vi "Begin.vi"(11 "Image Size":T6=enum."160x120") -> (0 "error out":errorcluster)   [LabVIEW 2011]
doc: "Called before other user functions, this VI is expected to open initial I/O refnums, load in file data, and do all program initialization. Notice that the <B>error out</B> terminal is simply used for data flow. Wiring it to other structures or subVIs ensures that this VI runs first."
uses:
  <vilib>/Rock Robotics/WPI/Camera/WPI_CameraImageSize.ctl
  <vilib>/Rock Robotics/SystemInterfaces/Typedef/FPGA_TypedefDigitalModule.ctl
  <vilib>/Rock Robotics/SystemInterfaces/CounterEncoderSourceConvertion/FPGA_CounterEncoderSourceConvertionLVSourceType.ctl
  <vilib>/Rock Robotics/SystemInterfaces/DIO/FPGA_DIODigitalSourceChannel.ctl
  <vilib>/Rock Robotics/SystemInterfaces/AnalogTrigger/FPGA_AnalogTriggerIndex.ctl
  <vilib>/Rock Robotics/SystemInterfaces/AnalogTrigger/FPGA_AnalogTriggerOutType.ctl
  <vilib>/Rock Robotics/WPI/Joystick/WPI_JoystickDeviceEnum.ctl
  <vilib>/Rock Robotics/WPI/Camera/WPI_CameraWhite Balance Values.ctl
  <vilib>/Rock Robotics/WPI/Camera/WPI_CameraExposure Values.ctl
  <vilib>/Rock Robotics/WPI/Camera/WPI_CameraFrameRate.ctl
  <vilib>/Rock Robotics/SystemInterfaces/DIO/FPGA_DIOPWMChannel.ctl
  <vilib>/Rock Robotics/WPI/Solenoid/WPI_SolenoidChannel.ctl
  <vilib>/Rock Robotics/SystemInterfaces/DIO/FPGA_DIORelayChannel.ctl
  <vilib>/Rock Robotics/SystemInterfaces/DIO/FPGA_DIOChannel.ctl
  <vilib>/Rock Robotics/SystemInterfaces/AI/FPGA_AIChannel.ctl
  <vilib>/Rock Robotics/WPI/Encoder/WPI_EncoderType.ctl
  <vilib>/Rock Robotics/WPI/RobotDrive/WPI_RobotDriveOpen2MotorWithVictor.vi
  <vilib>/Rock Robotics/WPI/Solenoid/WPI_SolenoidOpenSingle.vi
  <vilib>/Rock Robotics/WPI/Compressor/WPI_CompressorGetSetRefNum.vi
panel:
  in  "BSource 2":T1={"DevStatus"={"status"=FALSE, "code"=0, "source"=""}, "AnalogTriggerMode?"=FALSE, "DigitalMode"={"Digital Module"=enum."Digital Module 1", "DIO Channel"=enum."Disabled"}, "AnalogTriggerMode"={"AnalogTriggerIndex"=enum."Trig 0", "OutputType"=enum."InWindow"}}
  in  "ASource 2":T1={"DevStatus"={"status"=FALSE, "code"=0, "source"=""}, "AnalogTriggerMode?"=FALSE, "DigitalMode"={"Digital Module"=enum."Digital Module 1", "DIO Channel"=enum."Disabled"}, "AnalogTriggerMode"={"AnalogTriggerIndex"=enum."Trig 0", "OutputType"=enum."InWindow"}}
  in  "BSource":T1={"DevStatus"={"status"=FALSE, "code"=0, "source"=""}, "AnalogTriggerMode?"=FALSE, "DigitalMode"={"Digital Module"=enum."Digital Module 1", "DIO Channel"=enum."Disabled"}, "AnalogTriggerMode"={"AnalogTriggerIndex"=enum."Trig 0", "OutputType"=enum."InWindow"}}
  in  "ASource":T1={"DevStatus"={"status"=FALSE, "code"=0, "source"=""}, "AnalogTriggerMode?"=FALSE, "DigitalMode"={"Digital Module"=enum."Digital Module 1", "DIO Channel"=enum."Disabled"}, "AnalogTriggerMode"={"AnalogTriggerIndex"=enum."Trig 0", "OutputType"=enum."InWindow"}}
  in  "Pressure Switch Digital Module (Module 1)":T2
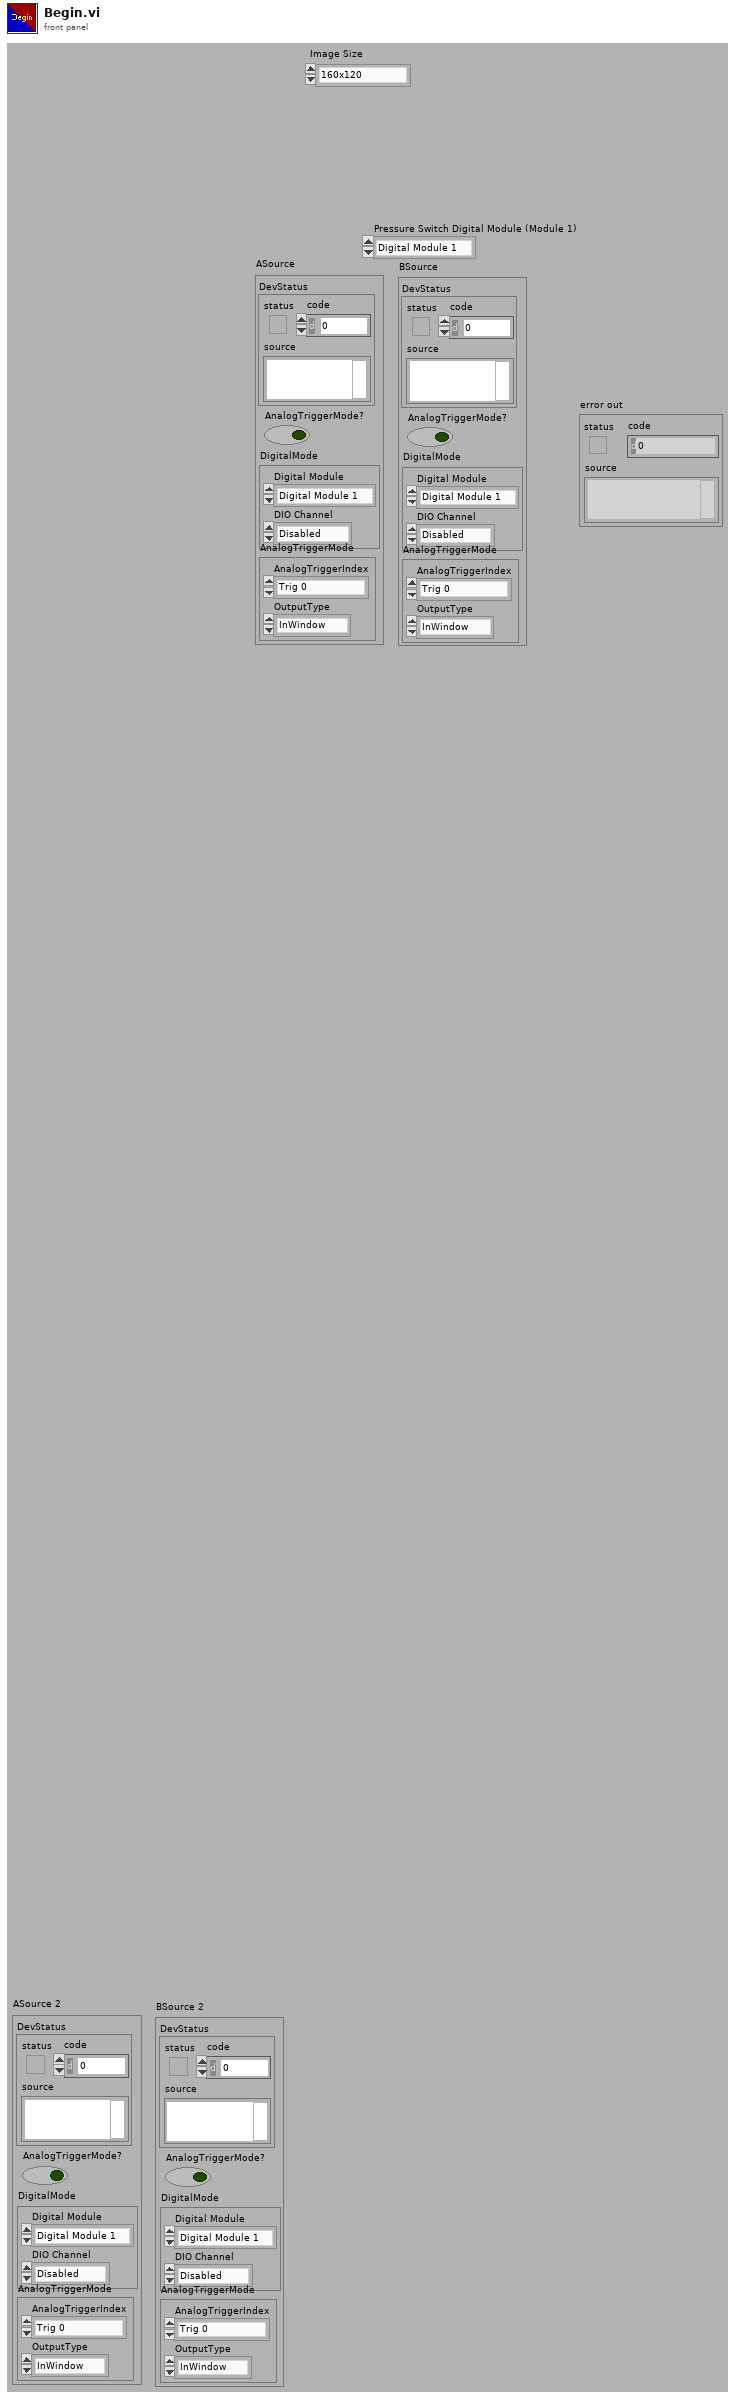
[diagram p1: front panel]
types:
  T1 = typedef "FPGA_CounterEncoderSourceConvertionLVSourceType.ctl" = cluster{"DevStatus":errorcluster, "AnalogTriggerMode?":bool, "DigitalMode":cluster{"Digital Module":T2, "DIO Channel":T3}, "AnalogTriggerMode":cluster{"AnalogTriggerIndex":T4, "OutputType":T5}}
  T2 = typedef "FPGA_TypedefDigitalModule.ctl" = enum16{"Digital Module 1", "Digital Module 2"}
  T3 = typedef "FPGA_DIODigitalSourceChannel.ctl" = enum8{"DIO 1", "DIO 2", "DIO 3", "DIO 4", "DIO 5", "DIO 6", "DIO 7", "DIO 8", "DIO 9", "DIO 10", "DIO 11", "DIO 12", "DIO 13", "DIO 14", "Disabled"}
  T4 = typedef "FPGA_AnalogTriggerIndex.ctl" = enum8{"Trig 0", "Trig 1", "Trig 2", "Trig 3", "Trig 4", "Trig 5", "Trig 6", "Trig 7", "Invalid"}
  T5 = typedef "FPGA_AnalogTriggerOutType.ctl" = enum16{"InWindow", "TriggerState", "Rising", "Falling"}
  T6 = typedef "WPI_CameraImageSize.ctl" = enum16{"640x480", "320x240", "160x120"}
  T7 = typedef "WPI_EncoderType.ctl" = enum16{"1x", "2x", "4x"}
  T8 = typedef "FPGA_DIOPWMChannel.ctl" = enum8{"PWM 1", "PWM 2", "PWM 3", "PWM 4", "PWM 5", "PWM 6", "PWM 7", "PWM 8", "PWM 9", "PWM 10", "Invalid"}
  T9 = typedef "FPGA_AIChannel.ctl" = enum8{"AI 1", "AI 2", "AI 3", "AI 4", "AI 5", "AI 6", "AI 7", "AI 8", "Invalid"}
  T10 = typedef "WPI_SolenoidChannel.ctl" = enum8{"Solenoid 1", "Solenoid 2", "Solenoid 3", "Solenoid 4", "Solenoid 5", "Solenoid 6", "Solenoid 7", "Solenoid 8", "Invalid"}
  T11 = typedef "FPGA_DIOChannel.ctl" = enum8{"DIO 1", "DIO 2", "DIO 3", "DIO 4", "DIO 5", "DIO 6", "DIO 7", "DIO 8", "DIO 9", "DIO 10", "DIO 11", "DIO 12", "DIO 13", "DIO 14", "Invalid"}
  T12 = typedef "FPGA_DIORelayChannel.ctl" = enum8{"Relay 1", "Relay 2", "Relay 3", "Relay 4", "Relay 5", "Relay 6", "Relay 7", "Relay 8", "Invalid"}
  T13 = typedef "WPI_JoystickDeviceEnum.ctl" = enum16{"USB 1", "USB 2", "USB 3", "USB 4", "Kinect 1", "Kinect 2"}
  T14 = typedef "WPI_CameraFrameRate.ctl" = u32
  T15 = typedef "WPI_CameraExposure Values.ctl" = enum16{"Auto", "Flicker-free 50 Hz", "Flicker-free 60 Hz", "Hold current"}
  T16 = typedef "WPI_CameraWhite Balance Values.ctl" = enum16{"Auto", "Fixed indoor", "Fixed outdoor 1", "Fixed outdoor 2", "Fixed fluorescent 1", "Fixed fluorescent 2", "Hold current"}
  T17 = typedef "WPI_AnalogChannelDevRef.ctl" = cluster{"DevStatus":errorcluster, "Analog Module":T18, "Analog Channel":T9}
  T18 = typedef "FPGA_TypedefAnalogModule.ctl" = enum16{"Analog Module 1", "Analog Module 2"}
  T19 = typedef "WPI_JoystickDevRef.ctl" = cluster{"Device":T13}
  T20 = typedef "WPI_SolenoidDevRef.ctl" = cluster{"DevStatus":errorcluster, "Solenoid Module":T21, "Forward Solenoid Channel":T10, "Reverse Solenoid Channel":T10}
  T21 = typedef "FPGA_TypedefSolenoidModule.ctl" = enum16{"Solenoid Module 1", "Solenoid Module 2"}
  T22 = typedef "WPI_CameraDevRef.ctl" = cluster{"Camera Address":string, "CameraStatus":errorcluster, "Acquire Image Notifier":refnum<notifier>}
  T23 = typedef "WPI_RobotDriveDevRef.ctl" = cluster{"DevStatus":errorcluster, "Motors[]":T24[], "Square Inputs":bool, "Max Output":dbl, "Isochronous":bool}
  T24 = typedef "WPI_MotorControlDeviceRef.ctl" = cluster{"DeviceStatus":errorcluster, "Type":enum16{"PWM", "CAN"}, "PWM":cluster{"Digital Module":T2, "PWM Channel":T8, "DeadBand":T25}, "CAN":cluster{"Device Number":u8, "Control Mode":T26, "Semaphore":T27, "Max Vout":dbl}, "Invert":bool, "TransformRef":T28, "InvTransformRef":T28}
  T25 = typedef "WPI_PWMDeadband.ctl" = cluster{"Name":string, "maxPositivePwm":i32, "minPositivePwm":i32, "centerPwm":i32, "maxNegativePwm":i32, "minNegativePwm":i32, "angularRange":u16}
  T26 = typedef "WPI_CANJaguar_ControlMode.ctl" = enum8{"Percent VBus", "Current", "Speed", "Position", "Voltage"}
  T27 = typedef "Semaphore RefNum" = refnum<k1>
  T28 = typedef "WPI_PWMTransform_ConPane.ctl" = refnum<vi>
  T29 = typedef "WPI_EncoderDevRef.ctl" = cluster{"DevStatus":errorcluster, "EncoderIndex":T30, "CounterIndex":T31, "DistancePerCount":dbl, "Decoding Type":T7}
  T30 = typedef "FPGA_EncoderIdx.ctl" = enum8{"Enc 0", "Enc 1", "Enc 2", "Enc 3", "Invalid"}
  T31 = typedef "FPGA_CounterCtrSystemIndex.ctl" = enum8{"Ctr 0", "Ctr 1", "Ctr 2", "Ctr 3", "Ctr 4", "Ctr 5", "Ctr 6", "Ctr 7", "Invalid"}
  T32 = typedef "WPI_CompressorDevRef.ctl" = cluster{"DevStatus":errorcluster, "DigitalInputDevRef":T33, "RelayDevRef":T34}
  T33 = typedef "WPI_DigitalInputDevRef.ctl" = cluster{"DevStatus":errorcluster, "DIO Channel":T11, "Digital Module":T2}
  T34 = typedef "WPI_RelayDevRef.ctl" = cluster{"DevStatus":errorcluster, "Relay Channel":T12, "Digital Module":T2, "Relay Direction":T35}
  T35 = typedef "WPI_RelayDirection.ctl" = enum16{"Both directions", "Forward only", "Reverse only"}
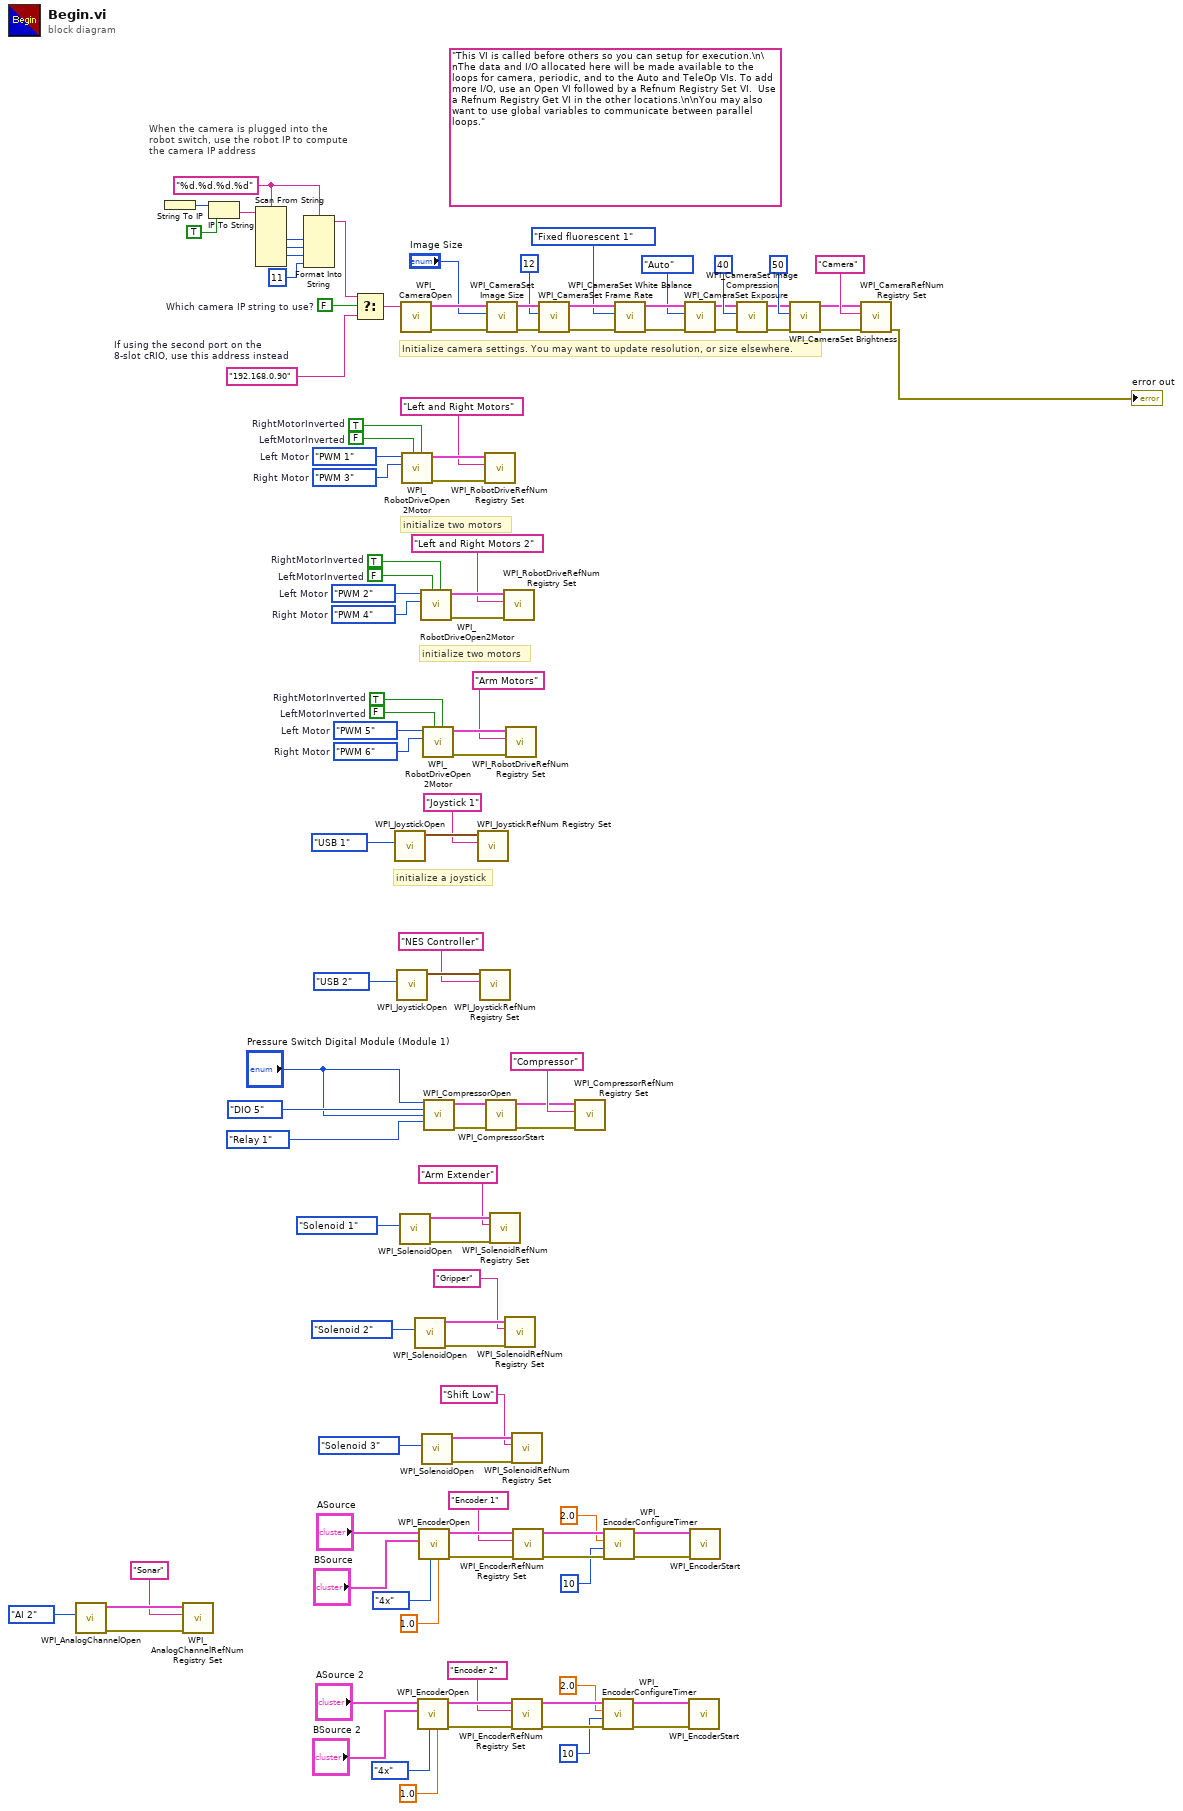
[diagram p0: block diagram]
diagram:
  w22 = FPGA_DIOPWMChannel."PWM 3"  # Right Motor
  w23 = FPGA_DIOPWMChannel."PWM 1"  # Left Motor
  w27 = FALSE  # LeftMotorInverted
  w28 = TRUE  # RightMotorInverted
  w29 = FPGA_DIOPWMChannel."PWM 4"  # Right Motor
  w30 = FPGA_DIOPWMChannel."PWM 2"  # Left Motor
  w34 = FALSE  # LeftMotorInverted
  w35 = TRUE  # RightMotorInverted
  w69 = FPGA_DIOPWMChannel."PWM 6"  # Right Motor
  w70 = FPGA_DIOPWMChannel."PWM 5"  # Left Motor
  w74 = FALSE  # LeftMotorInverted
  w75 = TRUE  # RightMotorInverted
  w76 = FALSE  # Which camera IP string to use?
  w80 = "%d.%d.%d.%d" ("format string")
  (unwired) "This VI is called before others so you can setup for execution.\n\nThe data and I/O allocated here will be made available to the loops for camera, periodic, and to the Auto and TeleOp VIs. To add more I/O, use an Open VI followed by a Refnum Registry Set VI.  Use a Refnum Registry Get VI in the other locations.\n\nYou may also want to use global variables to communicate between parallel loops."
  w77 = "192.168.0.90"  # If using the second port on the 8-slot cRIO, use this address instead
  # "initialize two motors"
  # "initialize two motors"
  # "When the camera is plugged into the\nrobot switch, use the robot IP to compute\nthe camera IP address"
  # "initialize a joystick"
  # "Initialize camera settings. You may want to update resolution, or size elsewhere."
  n1 = call <vilib>:"WPI_AnalogChannelOpen.vi"("Analog Channel"=FPGA_AIChannel."AI 2") -> ("error out"=w45:errorcluster, "AIDeviceRef"=w47:T17)  [unwired: 9 in]
  n2 = String To IP() -> (0:w87:u32)  [unwired: 1 in]
  n3 = call <vilib>:"WPI_AnalogChannelRefNum Registry Set.vi"("error in (no error)"=w45, "refnum name"="Sonar", "AIDeviceRef"=w47) -> ()  [unwired: 7 in, 2 out]
  n4 = IP To String(1:TRUE ("dot notation? (F)"), 2:w87) -> (0:w85:string)
  n5 = Scan From String(format string=w80, input string=w85) -> (output 1=w84:i32, output 2=w83:i32, output 3=w82:i32)  [unwired: 7 in, 3 out]
  n6 = Format Into String(format string=w80, w84, w83, w82, 11 ("Compression")) -> (resulting string=w78:string)  [unwired: 2 in, 1 out]
  n7 = Select(t=w78, s=w76, f=w77) -> (s? t:f=w79:string)
  n8 = call <vilib>:"WPI_JoystickOpen.vi"("JoystickDevice"=WPI_JoystickDeviceEnum."USB 1") -> ("JoystickDevRef"=w110:T19)  [unwired: 10 out]
  n9 = call <vilib>:"WPI_JoystickOpen.vi"("JoystickDevice"=WPI_JoystickDeviceEnum."USB 2") -> ("JoystickDevRef"=w68:T19)  [unwired: 10 out]
  n10 = call-poly <vilib>:"WPI_SolenoidOpen.vi"("Solenoid Channel"=WPI_SolenoidChannel."Solenoid 1") -> ("error out"=w54:errorcluster, "SolenoidDevRef"=w55:T20)  [unwired: 9 in]
  n11 = call <vilib>:"WPI_CameraOpen.vi"("Camera Address"=w79) -> ("error out"=w100:errorcluster, "CameraDevRef"=w101:T22)  [unwired: 1 in, 8 out]
  n12 = call-poly <vilib>:"WPI_RobotDriveOpen2Motor.vi"("Right Motor Inverted"=w28, "Left Motor Inverted"=w27, "Right Motor"=w22, "Left Motor"=w23) -> ("error out"=w24:errorcluster, "RobotDriveDevRef"=w26:T23)  [unwired: 1 in, 5 out]
  n13 = call-poly <vilib>:"WPI_SolenoidOpen.vi"("Solenoid Channel"=WPI_SolenoidChannel."Solenoid 2") -> ("error out"=w50:errorcluster, "SolenoidDevRef"=w51:T20)  [unwired: 9 in]
  n14 = call <vilib>:"WPI_EncoderOpen.vi"("DistancePerCount"=1.0, "Decoding Type"=WPI_EncoderType."4x", "BSource"="BSource 2", "ASource"="ASource 2") -> ("error out"=w8:errorcluster, "EncoderDevRef"=w9:T29)  [unwired: 6 in]
  n15 = call <vilib>:"WPI_EncoderOpen.vi"("DistancePerCount"=1.0, "Decoding Type"=WPI_EncoderType."4x", "BSource"="BSource", "ASource"="ASource") -> ("error out"=w38:errorcluster, "EncoderDevRef"=w39:T29)  [unwired: 6 in]
  n16 = call-poly <vilib>:"WPI_RobotDriveOpen2Motor.vi"("Right Motor Inverted"=w35, "Left Motor Inverted"=w34, "Right Motor"=w29, "Left Motor"=w30) -> ("error out"=w31:errorcluster, "RobotDriveDevRef"=w33:T23)  [unwired: 1 in, 5 out]
  n17 = call-poly <vilib>:"WPI_SolenoidOpen.vi"("Solenoid Channel"=WPI_SolenoidChannel."Solenoid 3") -> ("error out"=w64:errorcluster, "SolenoidDevRef"=w65:T20)  [unwired: 9 in]
  n18 = call-poly <vilib>:"WPI_RobotDriveOpen2Motor.vi"("Right Motor Inverted"=w75, "Left Motor Inverted"=w74, "Right Motor"=w69, "Left Motor"=w70) -> ("error out"=w71:errorcluster, "RobotDriveDevRef"=w73:T23)  [unwired: 1 in, 5 out]
  n19 = call <vilib>:"WPI_CompressorOpen.vi"("Pressure Switch Digital Module (Module 1)"="Pressure Switch Digital Module (Module 1)", "Pressure Switch DIO Channel"=FPGA_DIOChannel."DIO 5", "Relay Digital Module (Module 1)"="Pressure Switch Digital Module (Module 1)", "Relay Channel"=FPGA_DIORelayChannel."Relay 1") -> ("CompressorDevRef"=w61:T32, "error out"=w19:errorcluster)  [unwired: 10 in]
  n20 = call <vilib>:"WPI_JoystickRefNum Registry Set.vi"("refnum name"="Joystick 1", "JoystickDevRef"=w110) -> ()  [unwired: 1 in, 9 out]
  n21 = call <vilib>:"WPI_JoystickRefNum Registry Set.vi"("refnum name"="NES Controller", "JoystickDevRef"=w68) -> ()  [unwired: 1 in, 9 out]
  n22 = call <vilib>:"WPI_RobotDriveRefNum Registry Set.vi"("error in (no error)"=w24, "refnum name"="Left and Right Motors", "RobotDriveDevRef"=w26) -> ()  [unwired: 9 out]
  n23 = call <vilib>:"WPI_CompressorStart.vi"("error in (no error)"=w19, "CompressorDevRef"=w61) -> ("error out"=w20:errorcluster, "CompressorDevRef"=w60:T32)  [unwired: 8 in]
  n24 = call <vilib>:"WPI_CameraSet Image Size.vi"("error in (no error)"=w100, "Image Size"="Image Size", "CameraDevRef"=w101) -> ("error out"=w99:errorcluster, "CameraDevRef Out"=w102:T22)  [unwired: 7 out]
  n25 = call <vilib>:"WPI_SolenoidRefNum Registry Set.vi"("error in (no error)"=w54, "refnum name"="Arm Extender", "SolenoidDevRef"=w55) -> ()  [unwired: 7 in, 2 out]
  n26 = call <vilib>:"WPI_RobotDriveRefNum Registry Set.vi"("error in (no error)"=w31, "refnum name"="Left and Right Motors 2", "RobotDriveDevRef"=w33) -> ()  [unwired: 9 out]
  n27 = call <vilib>:"WPI_SolenoidRefNum Registry Set.vi"("error in (no error)"=w50, "refnum name"="Gripper", "SolenoidDevRef"=w51) -> ()  [unwired: 7 in, 2 out]
  n28 = call <vilib>:"WPI_RobotDriveRefNum Registry Set.vi"("error in (no error)"=w71, "refnum name"="Arm Motors", "RobotDriveDevRef"=w73) -> ()  [unwired: 9 out]
  n29 = call <vilib>:"WPI_SolenoidRefNum Registry Set.vi"("error in (no error)"=w64, "refnum name"="Shift Low", "SolenoidDevRef"=w65) -> ()  [unwired: 7 in, 2 out]
  n30 = call <vilib>:"WPI_EncoderRefNum Registry Set.vi"("error in (no error)"=w8, "refnum name"="Encoder 2", "EncoderDevRef"=w9) -> ("error out"=w4:errorcluster, "EncoderDevRef"=w6:T29)  [unwired: 7 in]
  n31 = call <vilib>:"WPI_EncoderRefNum Registry Set.vi"("error in (no error)"=w38, "refnum name"="Encoder 1", "EncoderDevRef"=w39) -> ("error out"=w17:errorcluster, "EncoderDevRef"=w21:T29)  [unwired: 7 in]
  n32 = call <vilib>:"WPI_CameraSet Frame Rate.vi"("error in (no error)"=w99, "Frame Rate (fps)"=T14 12, "CameraDevRef"=w102) -> ("error out"=w98:errorcluster, "CameraDevRef Out"=w104:T22)  [unwired: 7 out]
  n33 = call <vilib>:"WPI_CompressorRefNum Registry Set.vi"("error in (no error)"=w20, "refnum name"="Compressor", "CompressorDevRef"=w60) -> ()  [unwired: 7 in, 2 out]
  n34 = call <vilib>:"WPI_EncoderConfigureTimer.vi"("error in (no error)"=w4, "Number Samples to Average"=u8 10, "Minimum Rate"=2.0, "EncoderDevRef"=w6) -> ("error out"=w3:errorcluster, "EncoderDevRef"=w5:T29)  [unwired: 6 in]
  n35 = call <vilib>:"WPI_EncoderConfigureTimer.vi"("error in (no error)"=w17, "Number Samples to Average"=u8 10, "Minimum Rate"=2.0, "EncoderDevRef"=w21) -> ("error out"=w16:errorcluster, "EncoderDevRef"=w18:T29)  [unwired: 6 in]
  n36 = call <vilib>:"WPI_CameraSet White Balance.vi"("error in (no error)"=w98, "White Balance"=WPI_CameraWhite_Balance_Values."Fixed fluorescent 1", "CameraDevRef"=w104) -> ("error out"=w97:errorcluster, "CameraDevRef Out"=w103:T22)  [unwired: 7 out]
  n37 = call <vilib>:"WPI_CameraSet Exposure.vi"("error in (no error)"=w97, "Exposure"=WPI_CameraExposure_Values."Auto", "CameraDevRef"=w103) -> ("error out"=w96:errorcluster, "CameraDevRef Out"=w106:T22)  [unwired: 7 out]
  n38 = call <vilib>:"WPI_EncoderStart.vi"("error in (no error)"=w3, "EncoderDevRef"=w5) -> ()  [unwired: 8 in, 2 out]
  n39 = call <vilib>:"WPI_EncoderStart.vi"("error in (no error)"=w16, "EncoderDevRef"=w18) -> ()  [unwired: 8 in, 2 out]
  n40 = call <vilib>:"WPI_CameraSet Image Compression.vi"("error in (no error)"=w96, "Compression"=40, "CameraDevRef"=w106) -> ("error out"=w95:errorcluster, "CameraDevRef Out"=w105:T22)  [unwired: 7 out]
  n41 = call <vilib>:"WPI_CameraSet Brightness.vi"("error in (no error)"=w95, "Brightness"=50, "CameraDevRef"=w105) -> ("error out"=w93:errorcluster, "CameraDevRef Out"=w94:T22)  [unwired: 7 out]
  n42 = call <vilib>:"WPI_CameraRefNum Registry Set.vi"("error in (no error)"=w93, "refnum name"="Camera", "CameraDevRef"=w94) -> ("error out"=→"error out":errorcluster)  [unwired: 8 out]
